vi "Write Condition.vi"(10 "Allow":u16[](array[numeric]), 11 "IL U16 Allow in":refnum<class "IL U16 Pass.lvclass">) -> (3 "IL U16 Allow out":refnum<class "IL U16 Pass.lvclass">)   [LabVIEW 2015, in "Interlocks.lvlib" / "IL U16 Pass.lvclass"]
uses:
  IL U16 Pass.lvclass
  IL U16 Pass.lvclass/IL U16 Pass.ctl
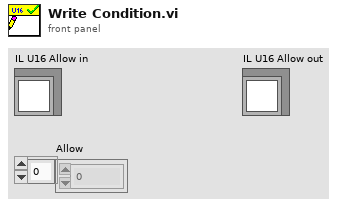
[diagram p1: front panel]
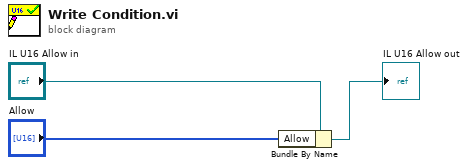
[diagram p0: block diagram]
diagram:
  n1 = Bundle By Name(cluster="IL U16 Allow in", "Allow"="Allow") -> (→"IL U16 Allow out":refnum<class "IL U16 Pass.lvclass">)
